vi "Read Attributes.vi"(11 "Set DER SetPointP Msg":refnum<class "Set DER SetPointP Msg.lvclass">) -> (2 "Payload":cluster{"DER_SetPointP":T1})   [LabVIEW 2018, in "Device Communication and Control Abstract Actor.lvlib" / "Set DER SetPointP Msg.lvclass"]
uses:
  Set DER SetPointP Msg.lvclass
  <vilib>/ORNL/CSEISMIC DDS/CSEISMIC DDS Base/Data Types/DER_SetPointP.ctl
  <vilib>/ORNL/CSEISMIC DDS/CSEISMIC DDS Base/Data Types/Controls/DeviceID.ctl
  Set DER SetPointP Msg.lvclass/Set DER SetPointP Msg.ctl
  <vilib>/ORNL/CSEISMIC DDS/CSEISMIC DDS Base/CSEISMIC DDS.lvclass
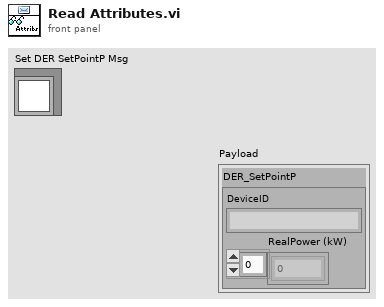
[diagram p1: front panel]
types:
  T1 = typedef "CSEISMIC DDS.lvlib/CSEISMIC DDS.lvclass/DER_SetPointP.ctl" = cluster{"DeviceID":T2, "RealPower (kW)":dbl[]}
  T2 = typedef "CSEISMIC DDS.lvlib/CSEISMIC DDS.lvclass/DeviceID.ctl" = string
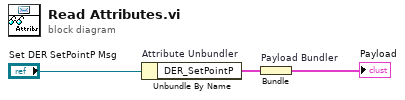
[diagram p0: block diagram]
diagram:
  n1 = Unbundle By Name "Attribute Unbundler"("Set DER SetPointP Msg") -> ("DER_SetPointP"=w1:T1)
  n2 = Bundle "Payload Bundler"("DER_SetPointP"=w1) -> (→"Payload":cluster{"DER_SetPointP":T1})  [unwired: 1 in]
